vi "Constructor.vi"(8 "error in (no error)":errorcluster, 10 "Table Name (Use Member Data)":string, 11 "Table Configuration Adv Schema DB in":refnum<class "Table Configuration Adv Schema DB.lvclass">) -> (0 "error out":errorcluster, 3 "Table Configuration Adv Schema DB out":refnum<class "Table Configuration Adv Schema DB.lvclass">)   [LabVIEW 2020, in "Table.lvlib" / "Table Configuration Adv Schema DB.lvclass"]
uses:
  Table Configuration Adv Schema DB.lvclass
  C:/Users/User/Desktop/Raman Program/Database OOP/source/Database OOP/Table Libraries/Basic Table/Configuration/Table Configuration Class/Table Configuration.lvclass
  Table Configuration Class/Table Configuration.lvclass/Table Configuration.ctl
  Table Configuration Adv Schema DB.lvclass/Table Configuration Adv Schema DB.ctl
  Column Libraries/Column Interface/FK Info.ctl
  Table Configuration Class/Table Configuration.lvclass
  Database Libraries/Database Interfaces/Database Advanced Schema Class/Database Adv Schema.lvclass
  Column Libraries/Column Interfaces.lvlib
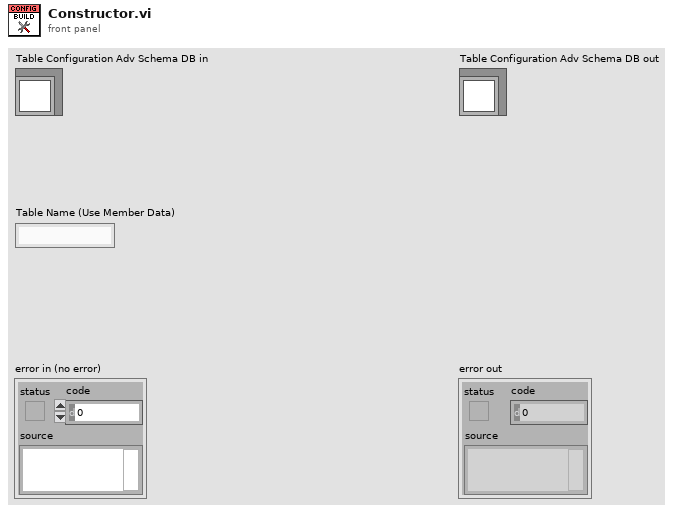
[diagram p1: front panel]
types:
  T1 = typedef "Column Interfaces.lvlib/FK Info.ctl" = cluster{"PK Table":string, "PK Column":string, "PK Display Column":string}
  T2 = typedef "Database Interfaces.lvlib/Primary Key Info.ctl" = cluster{"Primary Key Column":string, "Display Column":string}
  T3 = typedef "Database Interfaces.lvlib/foreign key properties.ctl" = cluster{"FK Table":string, "FK Column":string, "PK Table":string, "PK Column":string, "PK Display Column":string}
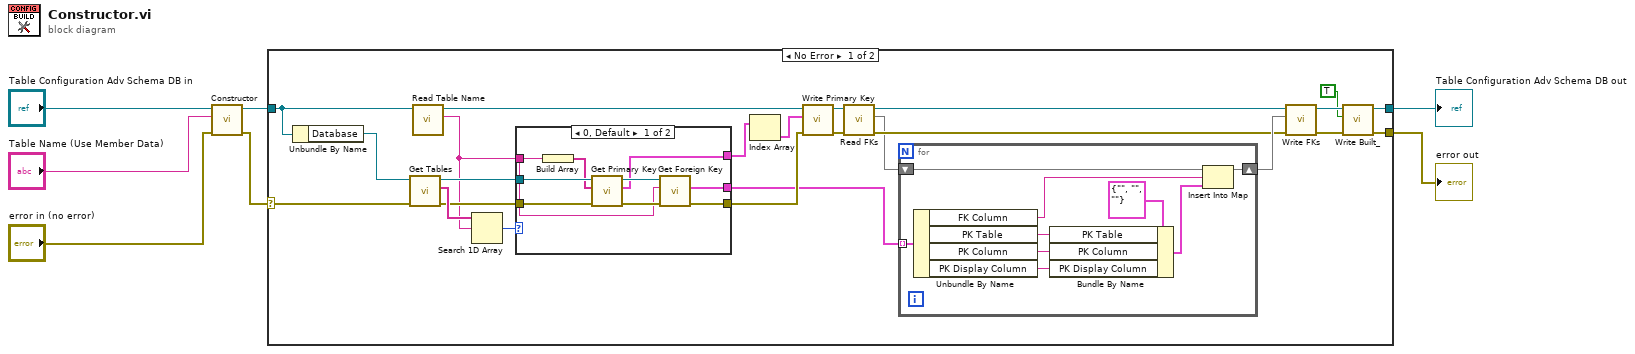
[diagram p0: block diagram]
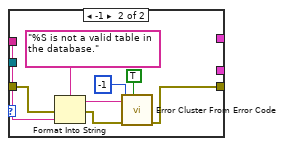
[diagram p2: hidden frame]
diagram:
  n1 = call-parent "Constructor.vi"("error in (no error)"="error in (no error)", "Table Name (Use Member Data)"="Table Name (Use Member Data)", "Table Configuration in"="Table Configuration Adv Schema DB in") -> ("error out"=w2:errorcluster, "Table Configuration out"=w5:refnum<class "Table Configuration Adv Schema DB.lvclass">)  [unwired: 7 in]
  n2 = case shown="No Error" w2 {
    selector: w2 -> [w25 w59]
    tunnel: [w17 w59] -> w3
    tunnel: [w16 w58] -> w4
    tunnel: w5 -> [w10 w58]
    frame No Error {
      n3 = Unbundle By Name(w10) -> ("Database"=w22:refnum<class "Database Adv Schema.lvclass">)
      n4 = call-dynamic "Get Tables.vi"("error in (no error)"=w25, "Database Interface in"=w22) -> ("error out"=w21:errorcluster, "Table Names"=w31:string[], "Database Interface out"=w29:refnum<class "Database Adv Schema.lvclass">)  [unwired: 7 in]
      n5 = call "Read Table Name.vi"("Table Configuration in"=w10) -> ("Table Name"=w8:string, "Table Configuration out"=w9:refnum<class "Table Configuration Adv Schema DB.lvclass">)  [unwired: 8 in, 1 out]
      n6 = Search 1D Array(1D array=w31, element=w8) -> (index of element=w30:i32)  [unwired: 1 in]
      n7 = case shown="0, Default" w30 {
        tunnel: w29 -> [w49 _]
        tunnel: w8 -> [w41 w57]
        tunnel: w21 -> [w47 w52]
        tunnel: [w42 w50] -> w26
        tunnel: [w44 _] -> w28
        tunnel: [w43 _] -> w24
        frame 0, Default {
          n8 = Build Array(w41) -> (w48:string[])
          n9 = call-dynamic "Get Primary Key.vi"("error in (no error)"=w47, "Table Name Array"=w48, "Database Schema in"=w49) -> ("error out"=w45:errorcluster, "Primary Key Array"=w44:T2[], "Database Schema out"=w46:refnum<class "Database Adv Schema.lvclass">)  [unwired: 5 in, 1 out]
          n10 = call-dynamic "Get Foreign Key.vi"("error in (no error)"=w45, "Table Name"=w41, "Database Advanced Schema in"=w46) -> ("error out"=w42:errorcluster, "FK Properties Array"=w43:T3[])  [unwired: 6 in, 1 out]
        }
        frame -1 {
          n11 = Format Into String(format string="%S is not a valid table in the database.", error in=w52, w57) -> (resulting string=w55:string, error out=w51:errorcluster)  [unwired: 1 in]
          n12 = call <vilib>:"Error Cluster From Error Code.vi"("show call chain? (False)"=TRUE, "error in (no error)"=w51, "error message (\"\")"=w55, "error code (0)"=-1) -> ("error out"=w50:errorcluster)  [unwired: 5 in]
        }
      }
      n13 = Index Array(array=w28) -> (element=w27:T2)  [unwired: 1 in]
      n14 = call "Write Primary Key.vi"("error in (no error)"=w26, "Primary Key"=w27, "Table Configuration in"=w9) -> ("error out"=w15:errorcluster, "Table Configuration out"=w11:refnum<class "Table Configuration Adv Schema DB.lvclass">)  [unwired: 7 in]
      n15 = call "Read FKs.vi"("error in (no error)"=w15, "Table Configuration in"=w11) -> ("error out"=w14:errorcluster, "FKs"=w12:map{string, T1}, "Table Configuration out"=w13:refnum<class "Table Configuration Adv Schema DB.lvclass">)  [unwired: 7 in]
      n16 = for {
        tunnel: w24 -> [w39] mode=indexing
        shift-right: [w32] -> w23
        shift-left: w12 -> [w40]
        n17 = Unbundle By Name(w39) -> ("FK Column"=w34:string, "PK Table"=w37:string, "PK Column"=w36:string, "PK Display Column"=w35:string)
        n18 = Bundle By Name(cluster=T1 {"PK Table"="", "PK Column"="", "PK Display Column"=""} ("value"), "PK Table"=w37, "PK Column"=w36, "PK Display Column"=w35) -> (w33:T1)
        n19 = Insert Into Map(map in=w40, key=w34, value=w33) -> (map out=w32:map{string, T1})  [unwired: 2 out]
      }
      n20 = call "Write FKs.vi"("error in (no error)"=w14, "FKs"=w23, "Table Configuration in"=w13) -> ("error out"=w18:errorcluster, "Table Configuration out"=w20:refnum<class "Table Configuration Adv Schema DB.lvclass">)  [unwired: 7 in]
      n21 = call "Write Built_.vi"("error in (no error)"=w18, "Built?"=TRUE, "Table Configuration in"=w20) -> ("error out"=w17:errorcluster, "Table Configuration out"=w16:refnum<class "Table Configuration Adv Schema DB.lvclass">)  [unwired: 7 in]
    }
    frame Error {
    }
  }
  "error out" <- w3
  "Table Configuration Adv Schema DB out" <- w4
